vi "Read alarm XML.vi"(0 "map in":T2) -> (7 "map out":T1, 8 "data":T3, 9 "change?":bool)   [LabVIEW 2016, in "Alarm interface.lvlib"]
uses:
  Alarm interface.lvlib
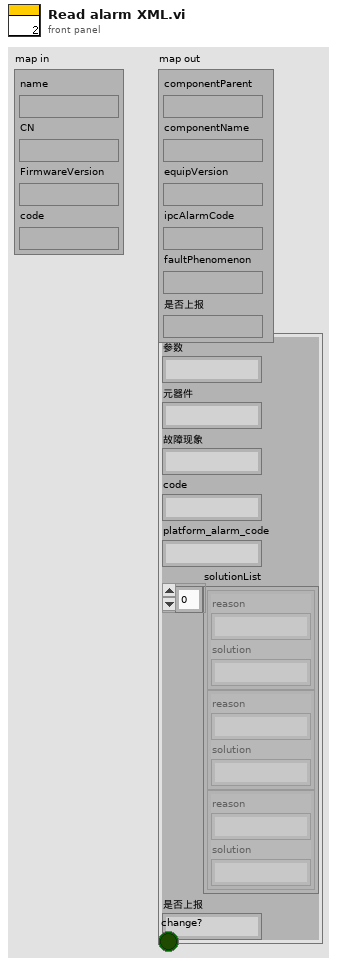
[diagram p1: front panel]
types:
  T1 = typedef "Alarm interface.lvlib/map out.ctl" = cluster{"componentParent":string, "componentName":string, "equipVersion":string, "ipcAlarmCode":string, "faultPhenomenon":string, "是否上报":string}
  T2 = typedef "Alarm interface.lvlib/map in.ctl" = cluster{"name":string, "CN":string, "FirmwareVersion":string, "code":string}
  T3 = typedef "Alarm interface.lvlib/报警短信语音交互.ctl" = cluster{"参数":string, "元器件":string, "故障现象":string, "code":string, "platform_alarm_code":string, "solutionList":cluster{"reason":string, "solution":string}[], "是否上报":string}
  T4 = cluster{"componentParentPath":string, "componentParentName":string, "componentName":string, "faultName":string, "equipVersion":string, "alarmCode":string, "ipcAlarmCode":string, "solutionList":cluster{"id":string, "faultId":string, "reason":string, "dataPhenomenon":string, "analysis":string, "solution":string}[]}
  T5 = cluster{"id":string, "faultId":string, "reason":string, "dataPhenomenon":string, "analysis":string, "solution":string}[]
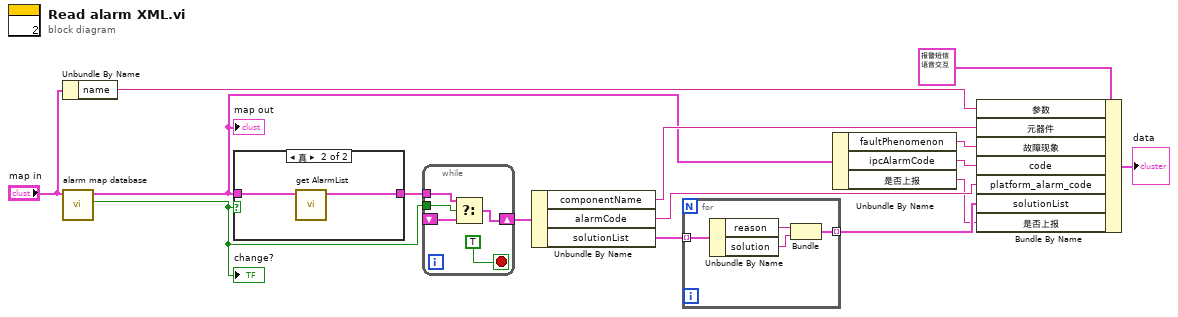
[diagram p0: block diagram]
diagram:
  n1 = Unbundle By Name("map in") -> ("name"=w6:string)
  n2 = call "alarm map database.vi"("map in"="map in") -> ("change?"=w8:bool, "map out"=w2:T1)  [unwired: 8 in, 1 out]
  "map out" <- w2
  "change?" <- w8
  n3 = case shown="真" w8 {
    tunnel: [_ w17] -> w14
    tunnel: w2 -> [_ w16]
    frame False {
    }
    frame True {
      n4 = call "get AlarmList.vi"("map out"=w16) -> ("alarm"=w17:T4)  [unwired: 9 in, 1 out]
    }
  }
  n5 = while {
    tunnel: w14 -> [w21]
    shift-right: [w19] -> w13
    shift-left: _ -> [w20]
    tunnel: w8 -> [w22]
    stop <- TRUE stop-if-true
    n6 = Select(t=w21, s=w22, f=w20) -> (s? t:f=w19:T4)
  }
  n7 = Unbundle By Name(w13) -> ("componentName"=w3:string, "alarmCode"=w12:string, "solutionList"=w11:T5)
  n8 = for {
    tunnel: w11 -> [w26] mode=indexing
    tunnel: [w23] -> w9 mode=indexing
    n9 = Unbundle By Name(w26) -> ("reason"=w25:string, "solution"=w24:string)
    n10 = Bundle("reason"=w25, "solution"=w24) -> (w23:cluster{"reason":string, "solution":string})  [unwired: 1 in]
  }
  n11 = Unbundle By Name(w2) -> ("faultPhenomenon"=w4:string, "ipcAlarmCode"=w5:string, "是否上报"=w1:string)
  n12 = Bundle By Name(cluster=T3 {"参数"="", "元器件"="", "故障现象"="", "code"="", "platform_alarm_code"="", "solutionList"=[{"reason"="1、缺标液，", "solution"="1、检查标液口（标液是否用完，及附属管路气密性等），检查管路气密性"}, {"reason"="2、液位传感器异常", "solution"="2、更换液位传感器"}, {"reason"="3、蠕动泵故障或泵管老化导致无法正常抽液", "solution"="3、更换蠕动泵管或更换蠕动泵"}], "是否上报"=""} ("data"), "参数"=w6, "元器件"=w3, "故障现象"=w4, "code"=w5, "platform_alarm_code"=w12, "solutionList"=w9, "是否上报"=w1) -> (→"data":T3)
